vi "ReadAllVirtualSetupClusterArray.vi"(8 "error in (no error)":errorcluster, 11 "VirtualOrigin.lvclass In":refnum<class "VirtualOrigin.lvclass">) -> (0 "error out":errorcluster, 2 "VirtualSetupClusterArray Out":T1 {"Y Step" min=1 step=1; "X Step" min=1 step=1}, 3 "VirtualOrigin.lvclass Out":refnum<class "VirtualOrigin.lvclass">)   [LabVIEW 2014, in "VirtualOrigin.lvclass"]
uses:
  VirtualOrigin.lvclass
  Project/VirtualSetupDataTypeDefine.ctl
  Control/AllVirtualTypeData.ctl
  VirtualOrigin.lvclass/VirtualOrigin.ctl
  Project/Project.lvclass
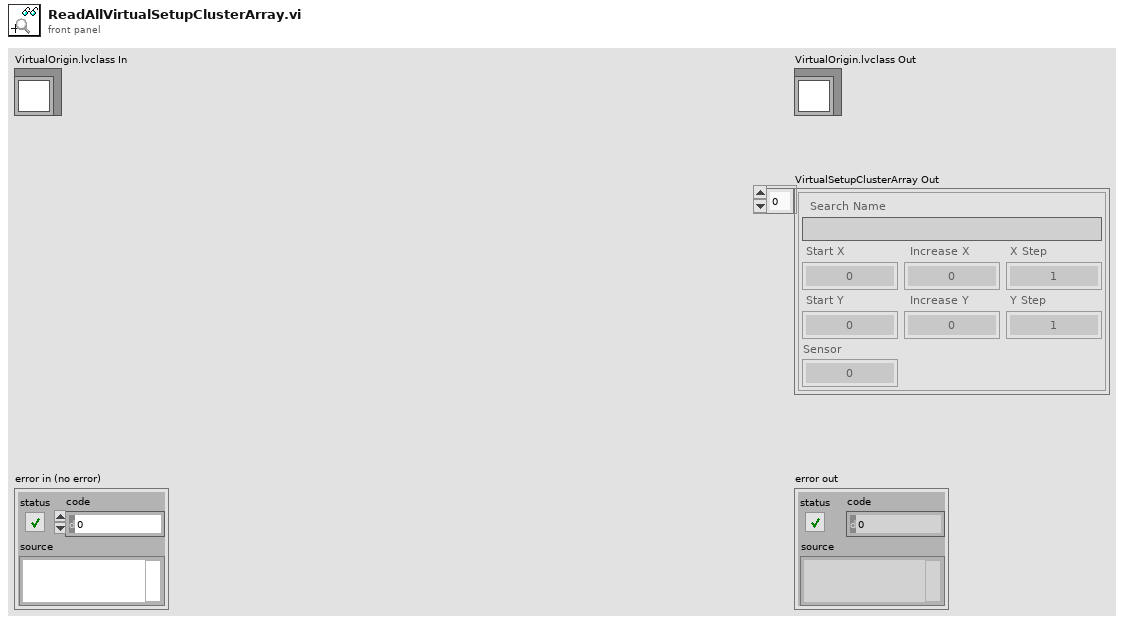
[diagram p1: front panel]
types:
  T1 = typedef "Project.lvclass/VirtualSetupDataTypeDefine.ctl" = T2[]
  T2 = typedef "VirtualOrigin.lvclass/AllVirtualTypeData.ctl" = cluster{"Search Name":string, "Start X":dbl, "Increase X":dbl, "X Step":i32, "Start Y":dbl, "Increase Y":dbl, "Y Step":i32, "Sensor":i32}
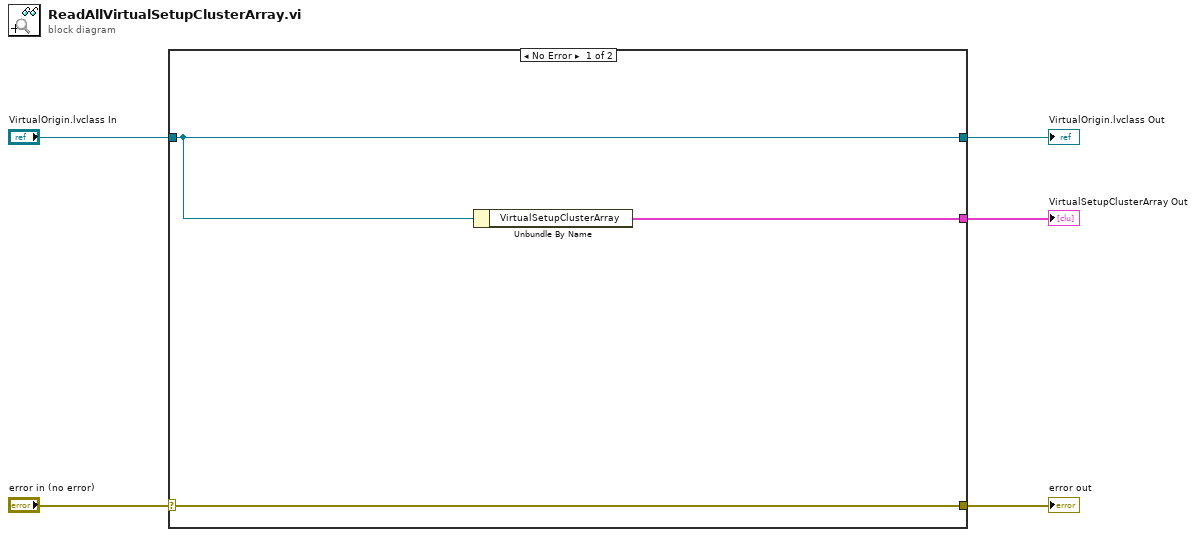
[diagram p0: block diagram]
diagram:
  n1 = case shown="No Error" "error in (no error)" {
    selector: "error in (no error)" -> [w8 w10]
    tunnel: [w8 w10] -> w4
    tunnel: "VirtualOrigin.lvclass In" -> [w7 w9]
    tunnel: [w7 w9] -> w2
    tunnel: [w6 _] -> w1
    frame No Error {
      n2 = Unbundle By Name(w7) -> ("VirtualSetupClusterArray"=w6:T1)
    }
    frame Error {
    }
  }
  "error out" <- w4
  "VirtualOrigin.lvclass Out" <- w2
  "VirtualSetupClusterArray Out" <- w1
